vi "convert32bit.vi"(1 "Array in":u32[](array[numeric])) -> (0 "Array out":u32[](array[numeric]))   [LabVIEW 2010]
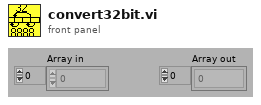
[diagram p1: front panel]
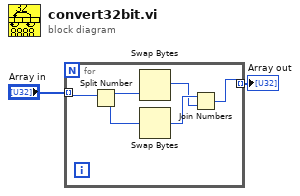
[diagram p0: block diagram]
diagram:
  n1 = for {
    tunnel: "Array in" -> [w5] mode=indexing
    tunnel: [w6] -> w2 mode=indexing
    n2 = Split Number(x=w5) -> (hi(x)=w8:u16, lo(x)=w7:u16)
    n3 = Swap Bytes(anything=w8) -> (byte swapped=w3:u16)
    n4 = Swap Bytes(anything=w7) -> (byte swapped=w4:u16)
    n5 = Join Numbers(hi=w4, lo=w3) -> ((hi.lo)=w6:u32)
  }
  "Array out" <- w2
